vi "NI Detection.vi"() -> (0 "NI 2":tag, 1 "NI 1":tag, 2 "Ok/Cancel":enum16{"Ok", "Cancel"}(ring))   [LabVIEW 2017]
uses:
  <resource>/objmgr/daqmx.rc
panel:
  in  "NI2":tag
  in  "NI1":tag
  in  "Cancel Button":bool
  in  "OK Button":bool
  # "PLease Choose Correct NI Serial Number"
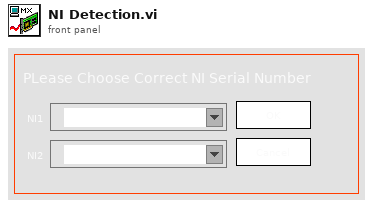
[diagram p1: front panel]
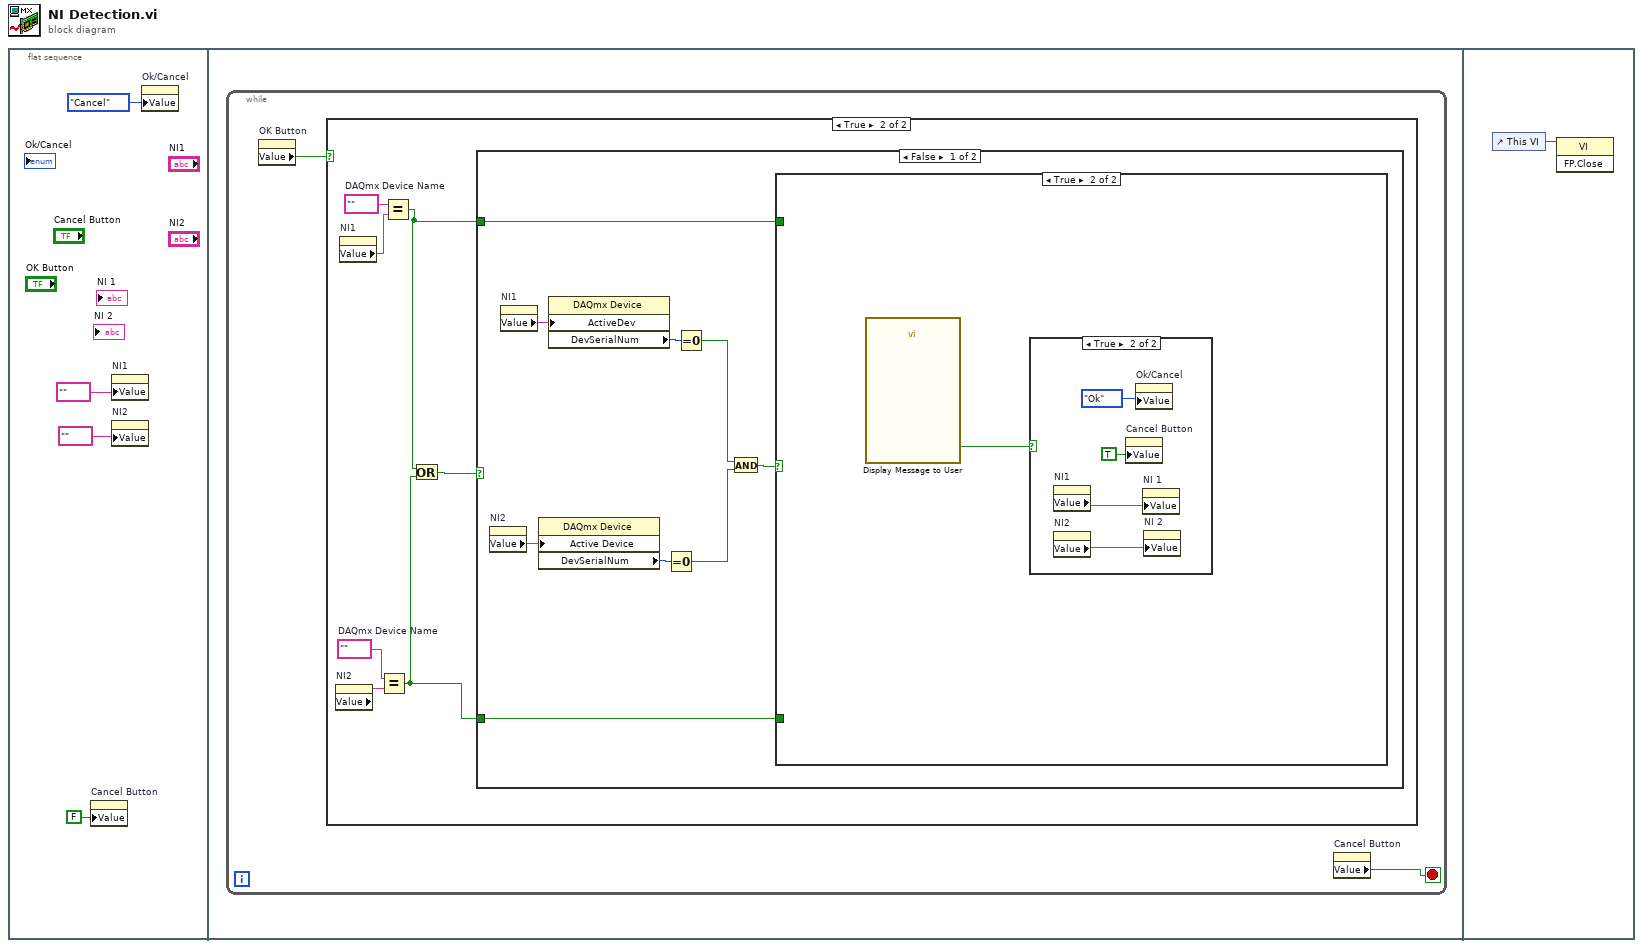
[diagram p0: block diagram]
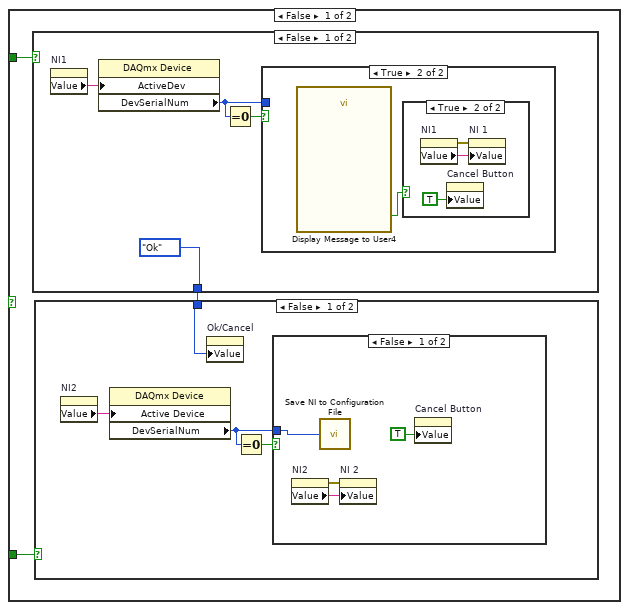
[diagram p3: hidden frame]
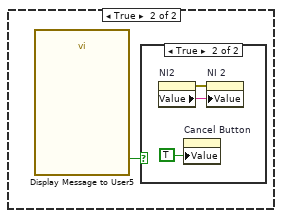
[diagram p4: hidden frame]
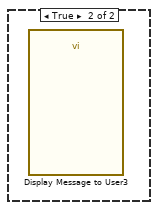
[diagram p6: hidden frame]
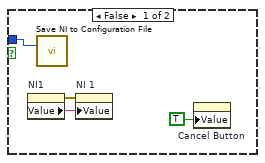
[diagram p7: hidden frame]
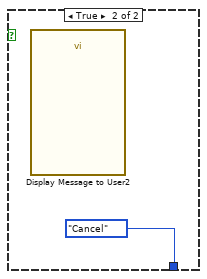
[diagram p9: hidden frame]
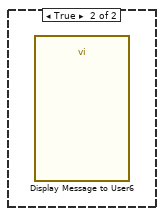
[diagram p11: hidden frame]
diagram:
  n1 = flat-sequence {
    frame #0 {
      n2 = property on="Cancel Button" class="Bool (strict)"("Value"=FALSE ("Cancel Button")) -> ()  [unwired: 2 in, 2 out]
      n3 = property on="NI1" class="DAQmxName"("Value"=tag "" ("NI 2")) -> ()  [unwired: 2 in, 2 out]
      n4 = property on="NI2" class="DAQmxName"("Value"=tag "" ("NI 2")) -> ()  [unwired: 2 in, 2 out]
      n5 = property on="Ok/Cancel" class="Enum (strict)"("Value"=enum16{"Ok", "Cancel"}."Cancel" ("Ok/Cancel")) -> ()  [unwired: 2 in, 2 out]
    }
    frame #1 {
      n6 = while {
        stop <- w5 stop-if-true
        n7 = property on="OK Button" class="Bool (strict)"() -> ("Value"=w6:bool)  [unwired: 2 in, 2 out]
        n8 = case shown="True" w6 {
          frame False {
          }
          frame True {
            w10 = tag ""  # DAQmx Device Name
            w13 = tag ""  # DAQmx Device Name
            n9 = property on="NI2" class="DAQmxName"() -> ("Value"=w11:string)  [unwired: 2 in, 2 out]
            n10 = property on="NI1" class="DAQmxName"() -> ("Value"=w12:string)  [unwired: 2 in, 2 out]
            n11 = Equal?(x=w10, y=w11) -> (x = y?=w7:bool)
            n12 = Equal?(x=w13, y=w12) -> (x = y?=w8:bool)
            n13 = Or(x=w8, y=w7) -> (x .or. y?=w9:bool)
            n14 = case shown="False" w9 {
              tunnel: w8 -> [w22 _]
              tunnel: w7 -> [w21 _]
              frame False {
                n15 = property on="NI2" class="DAQmxName"() -> ("Value"=w17:string)  [unwired: 2 in, 2 out]
                n16 = property on="NI1" class="DAQmxName"() -> ("Value"=w19:string)  [unwired: 2 in, 2 out]
                n17 = property class="DAQmx Device"("Active Device"=w17) -> ("DevSerialNum"=w18:u32)  [unwired: 2 in, 2 out]
                n18 = property class="DAQmx Device"("ActiveDev"=w19) -> ("DevSerialNum"=w20:u32)  [unwired: 2 in, 2 out]
                n19 = Equal To 0?(x=w18) -> (x = 0?=w15:bool)
                n20 = Equal To 0?(x=w20) -> (x = 0?=w16:bool)
                n21 = And(x=w16, y=w15) -> (x .and. y?=w14:bool)
                n22 = case shown="True" w14 {
                  tunnel: w22 -> [w25 _]
                  tunnel: w21 -> [w24 _]
                  frame False {
                    n23 = case shown="False" w25 {
                      tunnel: [enum16{"Ok", "Cancel"}."Ok" ("Ok/Cancel") enum16{"Ok", "Cancel"}."Cancel" ("Ok/Cancel")] -> w23
                      frame False {
                        n24 = property on="NI1" class="DAQmxName"() -> ("Value"=w41:string)  [unwired: 2 in, 2 out]
                        n25 = property class="DAQmx Device"("ActiveDev"=w41) -> ("DevSerialNum"=w39:u32)  [unwired: 2 in, 2 out]
                        n26 = Equal To 0?(x=w39) -> (x = 0?=w40:bool)
                        n27 = case shown="True" w40 {
                          tunnel: w39 -> [w42 _]
                          frame False {
                            n28 = property on="NI1" class="DAQmxName"() -> (error out=w45:errorcluster, "Value"=w44:string)  [unwired: 2 in, 1 out]
                            n29 = call "Save NI to Configuration File.vi"("NI1"=w42) -> ()  [unwired: 15 in]
                            n30 = property on="NI 1" class="DAQmxName"(error in=w45, "Value"=w44) -> ()  [unwired: 1 in, 2 out]
                            n31 = property on="Cancel Button" class="Bool (strict)"("Value"=TRUE ("Cancel Button")) -> ()  [unwired: 2 in, 2 out]
                          }
                          frame True {
                            n32 = call "Display Message to User4"() -> ("OK"=w46:bool)  [unwired: 10 in, 1 out]
                            n33 = case shown="True" w46 {
                              frame False {
                              }
                              frame True {
                                n34 = property on="NI1" class="DAQmxName"() -> (error out=w49:errorcluster, "Value"=w48:string)  [unwired: 2 in, 1 out]
                                n35 = property on="Cancel Button" class="Bool (strict)"("Value"=TRUE ("Cancel Button")) -> ()  [unwired: 2 in, 2 out]
                                n36 = property on="NI 1" class="DAQmxName"(error in=w49, "Value"=w48) -> ()  [unwired: 1 in, 2 out]
                              }
                            }
                          }
                        }
                      }
                      frame True {
                        n37 = call "Display Message to User2"() -> ()  [unwired: 10 in, 2 out]
                      }
                    }
                    n38 = case shown="False" w24 {
                      tunnel: w23 -> [w26 _]
                      frame False {
                        n39 = property on="NI2" class="DAQmxName"() -> ("Value"=w29:string)  [unwired: 2 in, 2 out]
                        n40 = property class="DAQmx Device"("Active Device"=w29) -> ("DevSerialNum"=w27:u32)  [unwired: 2 in, 2 out]
                        n41 = property on="Ok/Cancel" class="Enum (strict)"("Value"=w26) -> ()  [unwired: 2 in, 2 out]
                        n42 = Equal To 0?(x=w27) -> (x = 0?=w28:bool)
                        n43 = case shown="False" w28 {
                          tunnel: w27 -> [w30 _]
                          frame False {
                            n44 = property on="NI2" class="DAQmxName"() -> (error out=w33:errorcluster, "Value"=w32:string)  [unwired: 2 in, 1 out]
                            n45 = call "Save NI to Configuration File.vi"("NI2"=w30) -> ()  [unwired: 15 in]
                            n46 = property on="NI 2" class="DAQmxName"(error in=w33, "Value"=w32) -> ()  [unwired: 1 in, 2 out]
                            n47 = property on="Cancel Button" class="Bool (strict)"("Value"=TRUE ("Cancel Button")) -> ()  [unwired: 2 in, 2 out]
                          }
                          frame True {
                            n48 = call "Display Message to User5"() -> ("OK"=w34:bool)  [unwired: 10 in, 1 out]
                            n49 = case shown="True" w34 {
                              frame False {
                              }
                              frame True {
                                n50 = property on="NI2" class="DAQmxName"() -> (error out=w37:errorcluster, "Value"=w36:string)  [unwired: 2 in, 1 out]
                                n51 = property on="Cancel Button" class="Bool (strict)"("Value"=TRUE ("Cancel Button")) -> ()  [unwired: 2 in, 2 out]
                                n52 = property on="NI 2" class="DAQmxName"(error in=w37, "Value"=w36) -> ()  [unwired: 1 in, 2 out]
                              }
                            }
                          }
                        }
                      }
                      frame True {
                        n53 = call "Display Message to User3"() -> ()  [unwired: 10 in, 2 out]
                      }
                    }
                  }
                  frame True {
                    n54 = call "Display Message to User"() -> ("OK"=w51:bool)  [unwired: 10 in, 1 out]
                    n55 = case shown="True" w51 {
                      frame False {
                      }
                      frame True {
                        n56 = property on="NI1" class="DAQmxName"() -> ("Value"=w53:string)  [unwired: 2 in, 2 out]
                        n57 = property on="NI2" class="DAQmxName"() -> ("Value"=w52:string)  [unwired: 2 in, 2 out]
                        n58 = property on="Cancel Button" class="Bool (strict)"("Value"=TRUE ("Cancel Button")) -> ()  [unwired: 2 in, 2 out]
                        n59 = property on="Ok/Cancel" class="Enum (strict)"("Value"=enum16{"Ok", "Cancel"}."Ok" ("Ok/Cancel")) -> ()  [unwired: 2 in, 2 out]
                        n60 = property on="NI 1" class="DAQmxName"("Value"=w53) -> ()  [unwired: 2 in, 2 out]
                        n61 = property on="NI 2" class="DAQmxName"("Value"=w52) -> ()  [unwired: 2 in, 2 out]
                      }
                    }
                  }
                }
              }
              frame True {
                n62 = call "Display Message to User6"() -> ()  [unwired: 10 in, 2 out]
              }
            }
          }
        }
        n63 = property on="Cancel Button" class="Bool (strict)"() -> ("Value"=w5:bool)  [unwired: 2 in, 2 out]
      }
    }
    frame #2 {
      n64 = control-ref of="This VI"() -> (w56:refnum<vi>)
      n65 = invoke class="VI" method="FP.Close"(reference=w56) -> ()  [unwired: 2 in, 3 out]
    }
  }
